vi "SVC Sort Results.vi"   [LabVIEW 2017]
doc: "Sorts an array of peaks according to the <B>sort by</B> and <B>sort order</B> parameters. Use this VI to sort peaks that the SVFA Spectrum Peak Search, SVT Spurious Free Dynamic Range, and SVT THD and Harmonic Components VIs return. Wire data to the<B> peaks in</B> input to determine the polymorphic instance to use or manually select the instance."
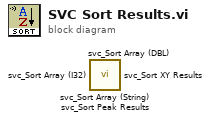
[diagram p0: block diagram]
diagram:
  n1 = call <vilib>:"svc_Sort Array (String).vi"() -> ()  [unwired: 10 in, 2 out]
  n2 = call <vilib>:"svc_Sort Array (DBL).vi"() -> ()  [unwired: 10 in, 2 out]
  n3 = call <vilib>:"svc_Sort Array (I32).vi"() -> ()  [unwired: 10 in, 2 out]
  n4 = call <vilib>:"svc_Sort XY Results.vi"() -> ()  [unwired: 10 in, 2 out]
  n5 = call <vilib>:"svc_Sort Peak Results.vi"() -> ()  [unwired: 10 in, 2 out]
